vi "LakeShore370 Set Heater.vi"(8 "error in (no error)":errorcluster, 10 "Heater range":T1, 11 "VISA resource name":refnum<visa-resource-name>) -> (0 "error out":errorcluster, 3 "VISA resource name out":refnum<visa-resource-name>)   [LabVIEW 2015]
uses:
  LakeShore370 Heater Ranges.ctl
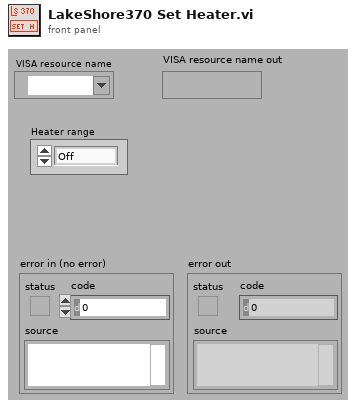
[diagram p1: front panel]
types:
  T1 = typedef "LakeShore370 Heater Ranges.ctl" = enum16{"Off", "31.6uA", "100uA", "316uA", "1mA", "3.16uA", "10mA", "31.6mA", "100mA"}
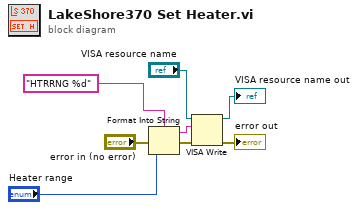
[diagram p0: block diagram]
diagram:
  n1 = Format Into String(format string="HTRRNG %d" ("data string in"), error in="error in (no error)", "Heater range") -> (resulting string=w7:string, error out=w5:errorcluster)  [unwired: 1 in]
  n2 = VISA Write(VISA resource name="VISA resource name", write buffer=w7, error in (no error)=w5) -> (VISA resource name out=→"VISA resource name out":refnum<visa-resource-name>, error out=→"error out":errorcluster)  [unwired: 1 out]
